vi "ArduPilot GCS.vi"() -> ()   [LabVIEW 8.6]
uses:
  user32.dll
  EventHandlerEnum.ctl
  Engines/SettingsEngine/SettingsEngineEnum.ctl
  EnumComm.ctl
  Engines/LogEngine/EnumLog.ctl
  Engines/SpeachEngine/EnumSpeak.ctl
panel:
  out "IMU":bool
  out "Climb Rate":dbl(knob) scale=-10.0..10.0 scale format="%#.2g"
  out "Mode":string
  out "WP":i32
  out "DistanceWP":i32 format="%.0f m"
  out "UAV Longitude":dbl format="%.6g°"
  out "UAV Latitude":dbl format="%.6g°"
  out "Throttle":i32(slide) scale=0.0..125.0
  out "Battery":dbl(slide) scale=0.0..10.0
  out "error outint comp manually":errorcluster
  out "error out clen-up":errorcluster
  in  "WebBrowser 2":refnum<k7>(container)
  in  "Heading":string="0"
  in  "Range":string="1000"
  in  "Tilt":string="0"
  in  "Send":bool
  in  "write buffer":string
  in  "Baud Rate":string(combo)="9600"
  in  "COM Port":refnum<visa-resource-name>
  out "Comm Status":bool
  in  "EARTHLib.IApplicationGE":refnum<k7>
  in  "EARTHLib.IKHInterface":refnum<k7>
  out "GPS fix":bool
  out "error out":errorcluster
  out "StatusMsg":string
  in  "Stop":bool
  in  "Tab Control":T1(tab)
  out "GndSpeed":i32(knob) scale=0.0..50.0
  out "AirSpeed":i32(knob) caption="Air Speed" scale=0.0..50.0
  out "Course   Bearing":cluster{i32, i32}(knob) scale=0.0..360.0 scale format="%.0f°"
  out "Altitude":cluster{i32, i32}(knob) scale=0.0..200.0
  out "Pitch":i32
  out "Roll":i32
  out "Roll Ind":cluster{i32, i32}(knob)={0, 180} scale=0.0..360.0
  out "Pitch-pic":picture
  in  "Zoom":u16(slide)=1000 scale=60000.0..1.0
  in  "Tilt":u8(slide) scale=0.0..90.0
  in  "Connect":bool
  in  "Baud Rate -M":string(combo)="9600"
  in  "COM Port -M":refnum<visa-resource-name>
  in  "kml write interval [s]":u32=1
  in  "Announcement interval [sec]":u32=30
  in  "Pan":i16(knob) scale=0.0..359.0
  out "IMU Performance data":string
  out "IMU health":i32
  out "Debug / Not Telemetry Data":string
  out "Raw Data":string
  # "%%%PWP:\t\t376322464,\t-1224913280,\t300,\nNWP:0,\t376321530,\t-1224913400,\t1200,***"
  # "Climb Rate"
  # "-122.491"
  # "37.6322"
  # "lon 122\nlat 37"
  # "meters"
  # "ALH"
  # "m / s"
  # "0"
  # "NOT USED"
  # "meters"
  # "meters"
  # "ALH"
  # "ALH"
  # "ALT"
  # "Gnd Speed"
  # "m/s"
  # "CRS"
  # "ASD"
  # "GSD"
  # "BER"
  # "AP port - manuall connection"
  # "To manually connect to AP serial port\nselect desired 'COM port' and 'Boud Rate' values\nand press 'Connect'"
  # "Google Earth Controls"
  # "Audio"
  # "N"
  # "(How often to update kml (GE) display)"
  # "Received"
  # "Set"
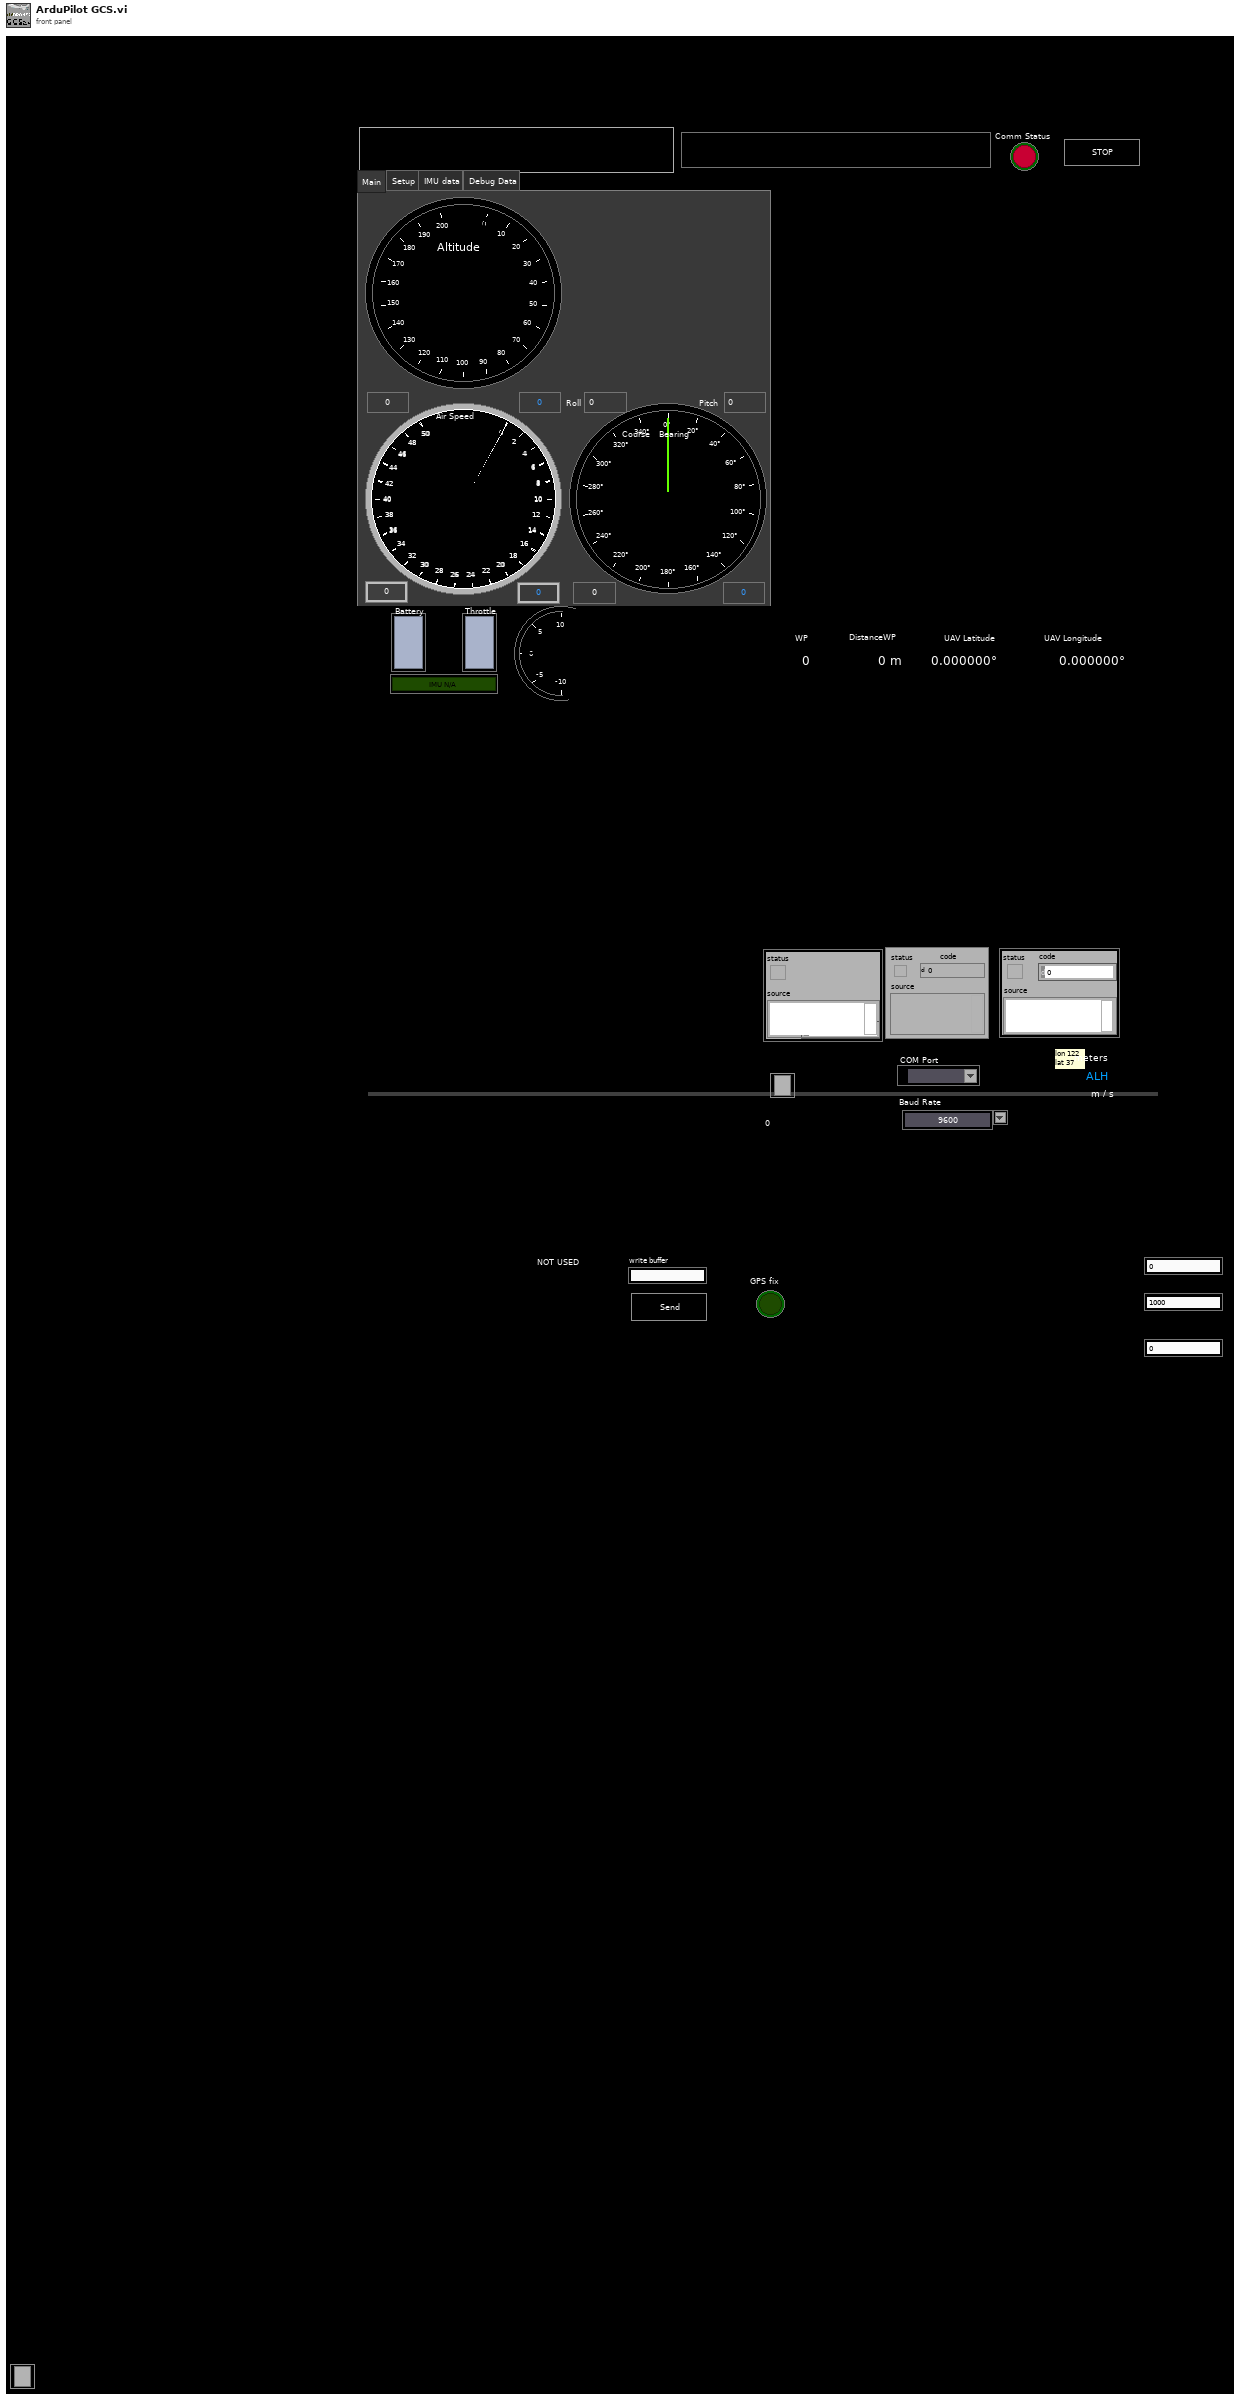
[diagram p1: front panel]
types:
  T1 = enum32{"Main", "Setup", "IMU data", "Debug Data"}
  T2 = typedef "EnumLog.ctl" = enum16{"Idle", "Log", "Init", "AddWP", "Stop", "CleanUp"}
  T3 = typedef "EnumComm.ctl" = enum16{"Read", "Idle", "Init", "InitComPort", "InitComPortManually", "Stop", "CleanUp", "Send"}
  T4 = typedef "EventHandlerEnum.ctl" = enum16{"Timeout", "Stop", "UpdateGEView", "UpdateCamData", "FPV_View_On", "UpdateIndicators"}
  T5 = typedef "EnumSpeak.ctl" = enum16{"Idle", "Init", "Speak", "Close"}
  T6 = cluster{"output number":i32, "output number":i32}
  T7 = typedef "SettingsEngineEnum.ctl" = enum16{"Init", "Load Settings from File", "Get Setting", "Set/Create Setting", "Save Settings to File"}
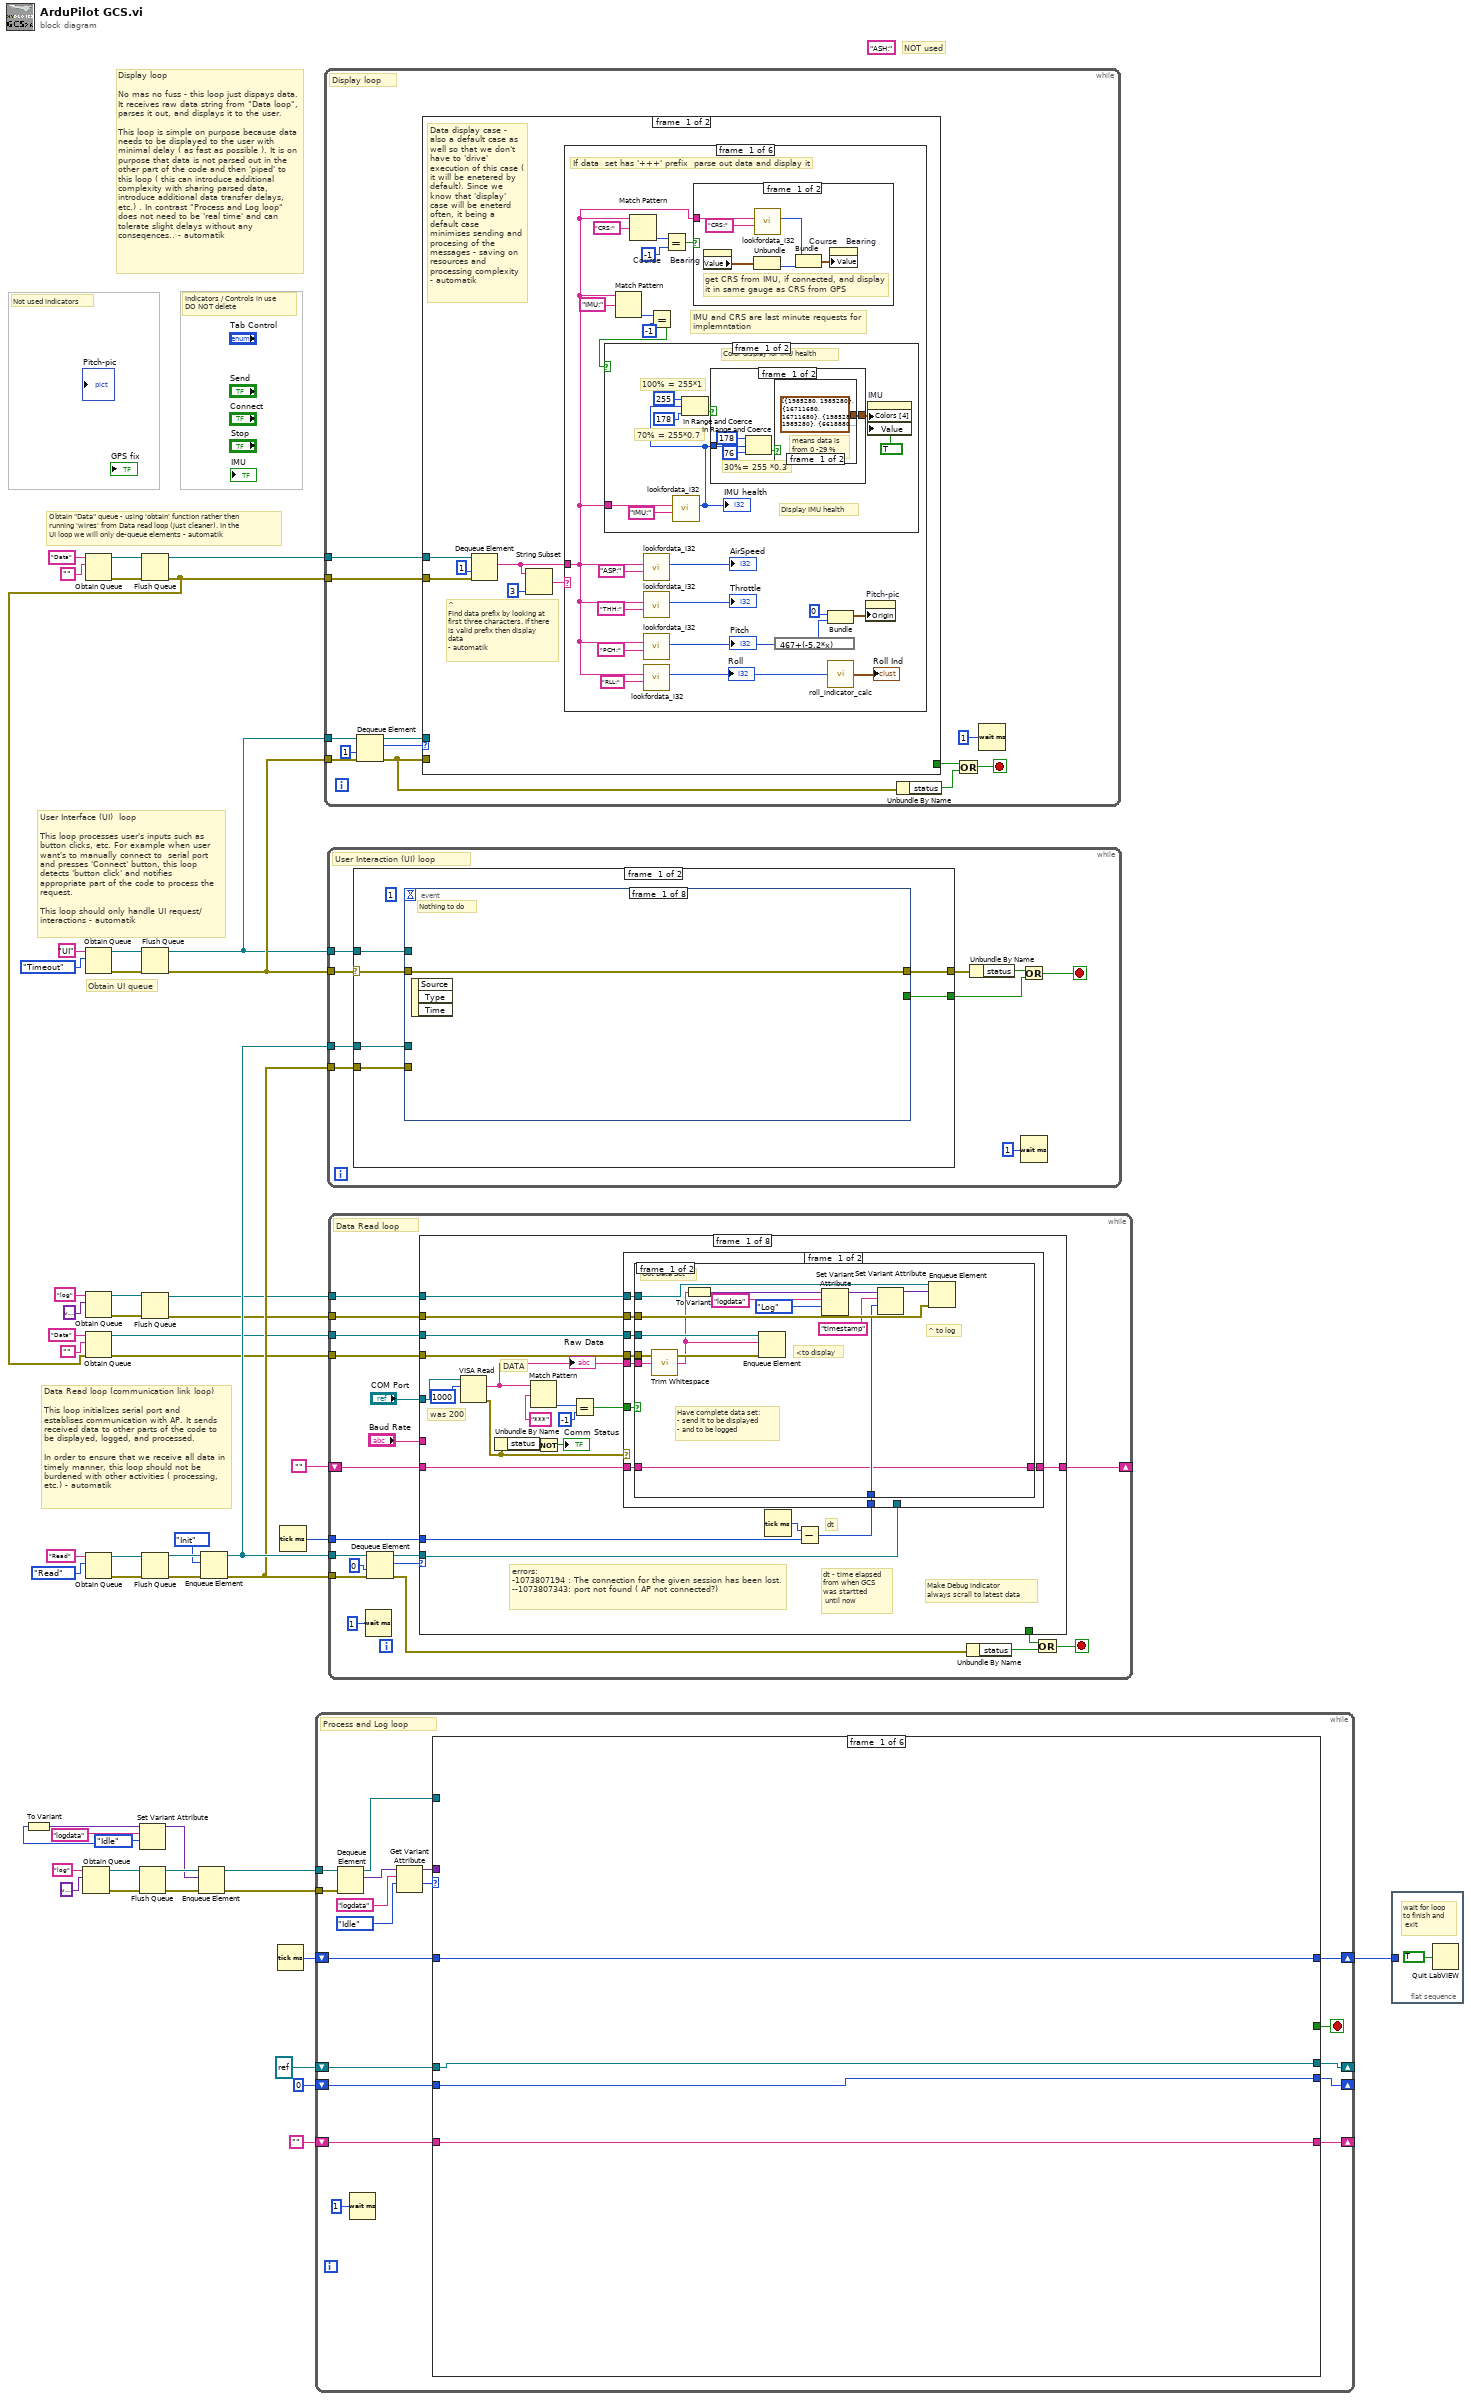
[diagram p0: block diagram]
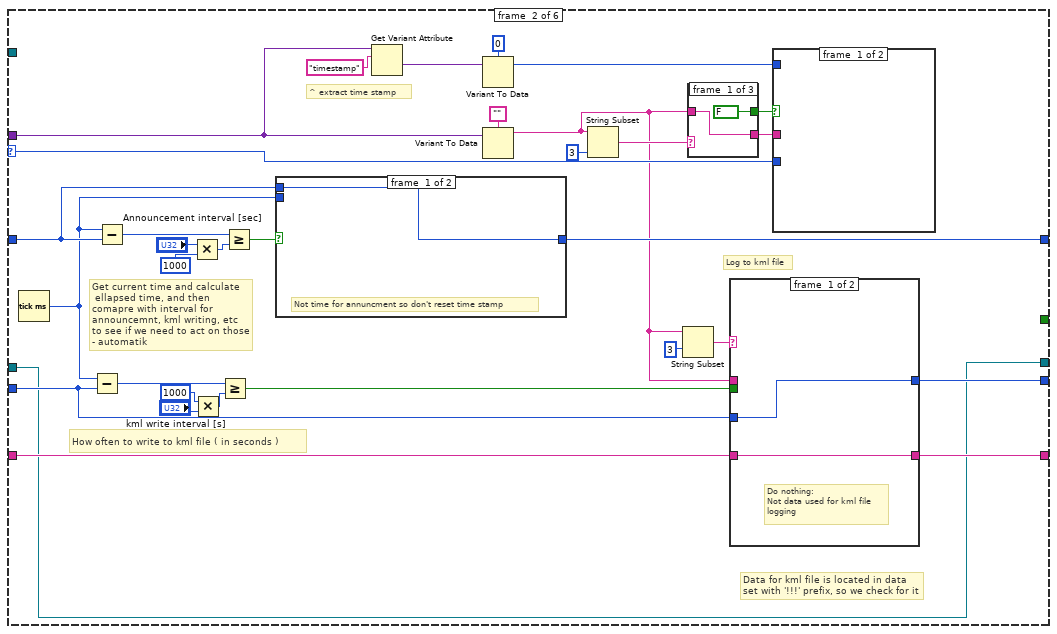
[diagram p2: hidden frame]
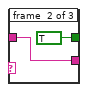
[diagram p3: hidden frame]
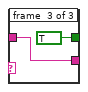
[diagram p4: hidden frame]
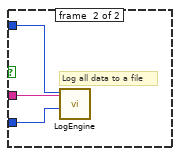
[diagram p5: hidden frame]
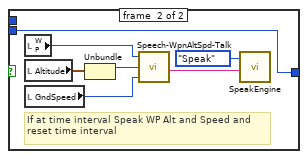
[diagram p6: hidden frame]
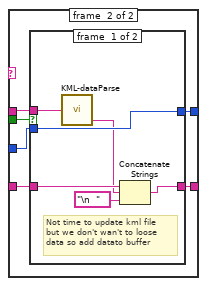
[diagram p7: hidden frame]
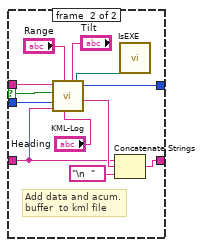
[diagram p8: hidden frame]
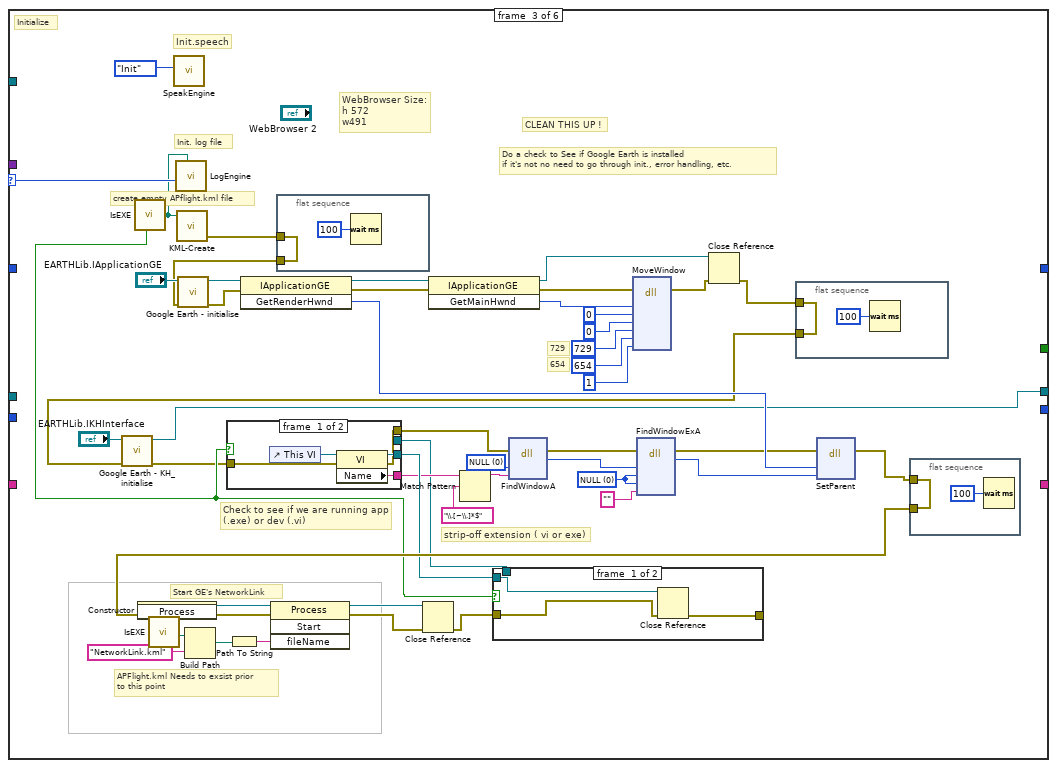
[diagram p9: hidden frame]
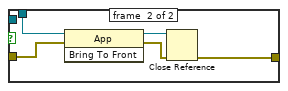
[diagram p10: hidden frame]
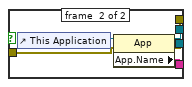
[diagram p11: hidden frame]
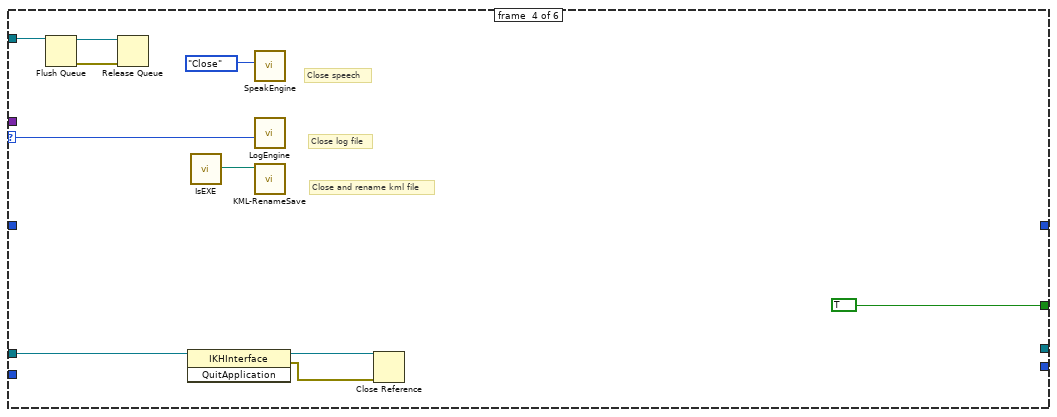
[diagram p12: hidden frame]
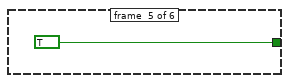
[diagram p13: hidden frame]
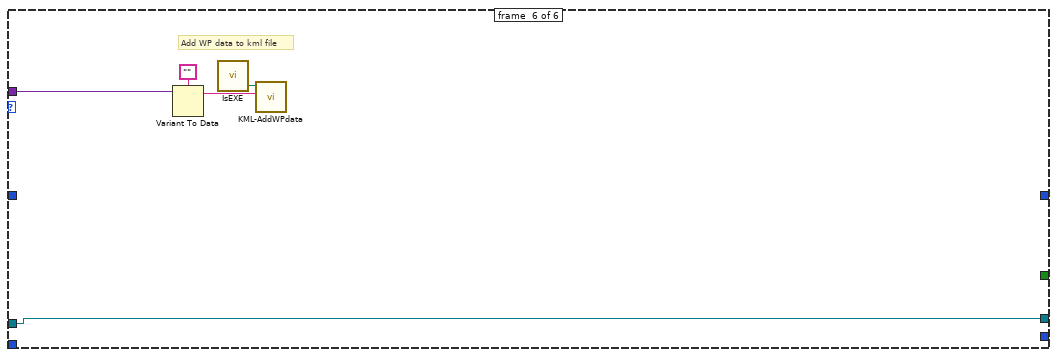
[diagram p14: hidden frame]
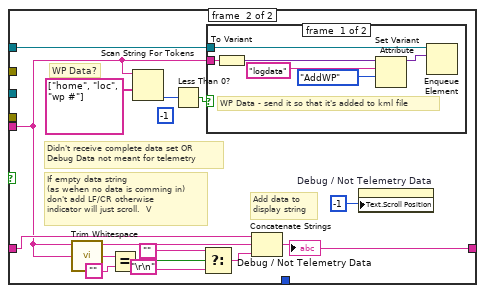
[diagram p15: hidden frame]
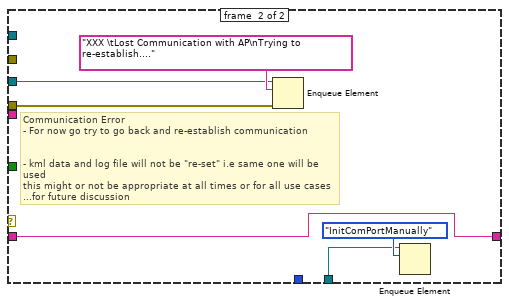
[diagram p17: hidden frame]
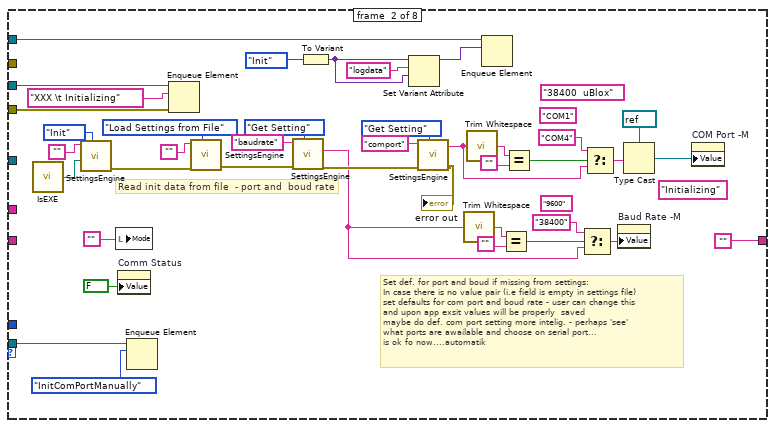
[diagram p18: hidden frame]
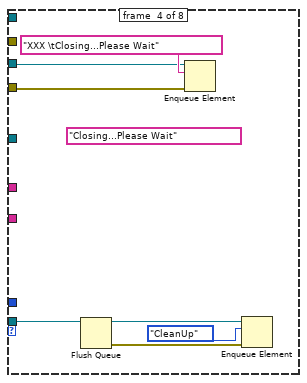
[diagram p20: hidden frame]
diagram:
  (unwired) "ASH:" ("regular expression")
  w12 = EnumLog."Idle" ("Log Enum")
  # "NOT used"
  # "Data Read loop (communication link loop)\n\nThis loop initializes serial port and establises communication with AP. It sends received data to other parts of the code to be displayed, logged, and processed.\n\nIn order to ensure that we receive all data in timely manner, this loop should not be burdened with other activities ( processing, etc.) - automatik"
  # "Obtain UI queue"
  # "User Interface (UI)  loop\n\nThis loop processes user's inputs such as button clicks, etc. For example when user want's to manually connect to  serial port and presses 'Connect' button, this loop detects 'button click' and notifies appropriate part of the code to process the request.\n\nThis loop should only handle UI request/ interactions - automatik"
  # "Obtain \"Data\" queue - using 'obtain' function rather then\nrunning 'wires' from Data read loop (just cleaner). In the\nUI loop we will only de-queue elements - automatik"
  # "Display loop\n\nNo mas no fuss - this loop just dispays data. It receives raw data string from \"Data loop\", parses it out, and displays it to the user. \n\nThis loop is simple on purpose because data needs to be displayed to the user with minimal delay ( as fast as possible ). It is on purpose that data is not parsed out in the other part of the code and then 'piped' to this loop ( this can introduce additional complexity with sharing parsed data, introduce additional data transfer delays, etc.) . In contrast \"Process and Log loop\"  does not need to be 'real time' and can tolerate slight delays without any conseqences.. - automatik"
  # "Indicators / Controls in use\nDO NOT delete"
  # "Not used indicators"
  n1 = To Variant(anything=w12) -> (Variant=w13:variant)
  n2 = Obtain Queue(name (unnamed)="log", element data type=variant ("variant")) -> (queue out=w19:refnum<queue>, error out=w7:errorcluster)  [unwired: 3 in, 1 out]
  n3 = Obtain Queue(name (unnamed)="Data", element data type="") -> (queue out=w29:refnum<queue>, error out=w27:errorcluster)  [unwired: 3 in, 1 out]
  n4 = Obtain Queue(name (unnamed)="UI", element data type=EventHandlerEnum."Timeout" ("Enum")) -> (queue out=w38:refnum<queue>, error out=w40:errorcluster)  [unwired: 3 in, 1 out]
  n5 = Obtain Queue(name (unnamed)="log", element data type=variant ("variant")) -> (queue out=w24:refnum<queue>, error out=w23:errorcluster)  [unwired: 3 in, 1 out]
  n6 = Obtain Queue(name (unnamed)="Read", element data type=EnumComm."Read" ("Comm Enum")) -> (queue out=w48:refnum<queue>, error out=w47:errorcluster)  [unwired: 3 in, 1 out]
  n7 = Set Variant Attribute(Variant=w13, name="logdata", value=w12) -> (Variant out=w11:variant)  [unwired: 1 in, 2 out]
  n8 = Flush Queue(queue=w19, error in (no error)=w7) -> (queue out=w16:refnum<queue>, error out=w5:errorcluster)  [unwired: 1 out]
  n9 = Flush Queue(queue=w29, error in (no error)=w27) -> (queue out=w28:refnum<queue>, error out=w26:errorcluster)  [unwired: 1 out]
  n10 = Obtain Queue(name (unnamed)="Data", element data type="", error in (no error)=w26) -> (queue out=w31:refnum<queue>, error out=w30:errorcluster)  [unwired: 2 in, 1 out]
  n11 = Flush Queue(queue=w38, error in (no error)=w40) -> (queue out=w37:refnum<queue>, error out=w39:errorcluster)  [unwired: 1 out]
  n12 = Flush Queue(queue=w24, error in (no error)=w23) -> (queue out=w22:refnum<queue>, error out=w21:errorcluster)  [unwired: 1 out]
  n13 = Flush Queue(queue=w48, error in (no error)=w47) -> (queue out=w46:refnum<queue>, error out=w45:errorcluster)  [unwired: 1 out]
  n14 = Enqueue Element(queue=w16, element=w11, error in (no error)=w5) -> (queue out=w15:refnum<queue>, error out=w4:errorcluster)  [unwired: 1 in, 1 out]
  n15 = Enqueue Element(queue=w46, element=EnumComm."Init" ("Comm Enum"), error in (no error)=w45) -> (queue out=w42:refnum<queue>, error out=w41:errorcluster)  [unwired: 1 in, 1 out]
  n16 = Tick Count (ms)() -> (millisecond timer value=w6:u32)
  n17 = Tick Count (ms)() -> (millisecond timer value=w10:u32)
  n18 = while {
    tunnel: w15 -> [w53]
    tunnel: w4 -> [w68]
    shift-right: [w61] -> _
    shift-left: "" -> [w60]
    shift-right: [w59] -> _
    shift-left: u32 0 ("millisecond timer value") -> [w58]
    shift-right: [w55] -> w2
    shift-left: w6 -> [w56]
    shift-right: [w52] -> _
    shift-left: refnum<k7> refnum ("Refnum Out") -> [w51]
    stop <- w63 stop-if-true
    # "Process and Log loop"
    n19 = Dequeue Element(queue=w53, error in (no error)=w68) -> (queue out=w54:refnum<queue>, element=w67:variant)  [unwired: 1 in, 2 out]
    n20 = Wait (ms)(milliseconds to wait=u32 1) -> ()  [unwired: 1 out]
    n21 = Get Variant Attribute(Variant=w67, name="logdata", default value (empty Variant)=EnumLog."Idle" ("Log Enum")) -> (duplicate Variant=w64:variant, value=w65:T2)  [unwired: 1 in, 2 out]
    n22 = case shown="\"Init\"" w65 {
      selector: w65 -> [_ w94 w193 w230 _ _]
      tunnel: w64 -> [_ w103 _ _ _ w236]
      tunnel: [_ _ _ TRUE ("x") TRUE ("x") _] -> w63
      tunnel: [w71 w97 _ _ _ _] -> w61
      tunnel: w60 -> [w71 w96 _ _ _ _]
      tunnel: [w72 w95 _ _ _ _] -> w59
      tunnel: w58 -> [w72 w93 _ _ _ _]
      tunnel: w56 -> [w70 w82 _ _ _ _]
      tunnel: [w70 w80 _ _ _ _] -> w55
      tunnel: w54 -> [_ _ _ w226 _ _]
      tunnel: [w69 w73 w151 _ _ w233] -> w52
      tunnel: w51 -> [w69 w73 _ w224 _ w233]
      frame #0 {
      }
      frame #1 {
        # "Get current time and calculate\n ellapsed time, and then comapre with interval for announcemnt, kml writing, etc to see if we need to act on those - automatik"
        # "Data for kml file is located in data\nset with '!!!' prefix, so we check for it"
        # "^ extract time stamp"
        # "Log to kml file"
        # "How often to write to kml file ( in seconds )"
        n23 = Tick Count (ms)() -> (millisecond timer value=w81:u32)
        n24 = Subtract(x=w81, y=w93) -> (x-y=w98:u32)
        n25 = Subtract(x=w81, y=w82) -> (x-y=w84:u32)
        n26 = Multiply(x="Announcement interval [sec]", y=u32 1000) -> (x*y=w85:u32)
        n27 = Multiply(x=u32 1000, y="kml write interval [s]") -> (x*y=w89:u32)
        n28 = Greater Or Equal?(x=w98, y=w89) -> (x >= y?=w92:bool)
        n29 = Greater Or Equal?(x=w84, y=w85) -> (x >= y?=w83:bool)
        n30 = case shown="True" w83 {
          tunnel: w82 -> [w114 _]
          tunnel: w81 -> [_ w116]
          tunnel: [w114 w116] -> w80
          frame #0 {
            # "Not time for annuncment so don't reset time stamp"
          }
          frame #1 {
            # "If at time interval Speak WP Alt and Speed and reset time interval"
            n31 = local read "WP"() -> (w120:i32)
            n32 = local read "Altitude"() -> (w119:cluster{i32, i32})
            n33 = local read "GndSpeed"() -> (w115:i32)
            n34 = Unbundle(w119) -> (w121:i32)  [unwired: 1 out]
            n35 = call "Speech-WpnAltSpd-Talk.vi"("Ground Speed"=w115, "Altitude"=w121, "Current WP"=w120) -> ("Text"=w118:string)
            n36 = call "SpeakEngine.vi"("Text to speak"=w118, "EnumSpeak"=EnumSpeak."Speak") -> ()  [unwired: 9 in, 1 out]
          }
        }
        n37 = Get Variant Attribute(Variant=w103, name="timestamp") -> (value=w101:variant)  [unwired: 2 in, 3 out]
        n38 = Variant To Data(Variant=w101, type=u32 0 ("x-y 2")) -> (data=w99:u32)  [unwired: 1 in, 1 out]
        n39 = Variant To Data(Variant=w103, type="") -> (data=w75:string)  [unwired: 1 in, 1 out]
        n40 = String Subset(string=w75, length (rest)=3 ("length (rest)")) -> (substring=w76:string)  [unwired: 1 in]
        n41 = String Subset(string=w75, length (rest)=3 ("length (rest)")) -> (substring=w90:string)  [unwired: 1 in]
        n42 = case shown="\"+++\"" w76 {
          tunnel: [w105 w107 w109] -> w79
          tunnel: [FALSE TRUE TRUE] -> w78
          tunnel: w75 -> [w105 w107 w109]
          frame #0 {
          }
          frame #1 {
          }
          frame #2 {
          }
        }
        n43 = case shown="\"!!!\"" w90 {
          tunnel: [w122 w129] -> w97
          tunnel: w96 -> [w122 w128]
          tunnel: [w123 w127] -> w95
          tunnel: w93 -> [w123 w126]
          tunnel: w92 -> [_ w124]
          tunnel: w75 -> [_ w125]
          frame #0 {
            # "Do nothing:\nNot data used for kml file\nlogging"
          }
          frame #1 {
            n44 = case shown="True" w124 {
              selector: w124 -> [_ w139]
              tunnel: [w132 w146] -> w129
              tunnel: w128 -> [w133 w143]
              tunnel: [w134 w142] -> w127
              tunnel: w126 -> [w134 w141]
              tunnel: w125 -> [w131 w140]
              frame #0 {
                # "Not time to update kml file\nbut we don't wan't to loose\ndata so add datato buffer"
                n45 = call "KML-dataParse.vi"("data in"=w131) -> ("Cur loc (out)"=w130:string)  [unwired: 1 in, 1 out]
                n46 = Concatenate Strings(w133, w130, "\n  " ("string")) -> (w132:string)
              }
              frame #1 {
                # "Add data and acum. \nbuffer  to kml file"
                n47 = call "IsEXE.vi"() -> ("path to vi or exe install\\data\\ dir"=w145:path)  [unwired: 10 out]
                n48 = call "KML-Log.vi"("path to vi or exe (in)"=w145, "Tilt"="Tilt", "Heading"="Heading", "Range"="Range", "Coords (in)"=w143, "TimerIN (sh)"=w141, "WriteToFile?"=w139, "data in"=w140) -> ("Cur loc (out)"=w144:string, "Timer OUT (sh)"=w142:u32)  [unwired: 2 in]
                n49 = Concatenate Strings(w143, w144, "\n  " ("string")) -> (w146:string)
              }
            }
          }
        }
        n50 = case shown="True" w78 {
          tunnel: w99 -> [_ w113]
          tunnel: w94 -> [_ w112]
          tunnel: w79 -> [_ w111]
          frame #0 {
          }
          frame #1 {
            # "Log all data to a file"
            n51 = call "LogEngine.vi"("Log Enum"=w112, "LogDataIN"=w111, "cumul time"=w113) -> ()  [unwired: 9 in]
          }
        }
      }
      frame #2 {
        w181 = 0 items=["NULL"]
        w190 = 0 items=["NULL"]
        # "CLEAN THIS UP !"
        # "strip-off extension ( vi or exe)"
        # "Check to see if we are running app\n(.exe) or dev (.vi)"
        # "Do a check to See if Google Earth is installed\nif it's not no need to go through init., error handling, etc."
        # "create empty APflight.kml file"
        # "WebBrowser Size:\nh 572\nw491"
        # "729"
        # "654"
        # "APFlight.kml Needs to exsist prior\nto this point"
        # "Start GE's NetworkLink"
        # "Init.speech"
        # "Init. log file"
        # "Initialize"
        n52 = call "Google Earth - KH_initialise.vi"("error in (no error)"=w168, "EARTHLib.IKHInterface"="EARTHLib.IKHInterface") -> ("error out"=w152:errorcluster, "Refnum Out"=w151:refnum<k7>)  [unwired: 8 out]
        n53 = call "IsEXE.vi"() -> ("path to vi or exe install\\data\\ dir"=w163:path, "is exe?"=w161:bool)  [unwired: 9 out]
        n54 = constructor class="Process"(error in=w164) -> (reference out=w170:refnum<k24>, error out=w169:errorcluster)  [unwired: 2 in, 1 out]
        n55 = call "IsEXE.vi"() -> ("path to vi or exe install\\data\\ dir"=w195:path)  [unwired: 10 out]
        n56 = call "SpeakEngine.vi"("EnumSpeak"=EnumSpeak."Init") -> ()  [unwired: 10 in, 1 out]
        n57 = call "LogEngine.vi"("dir path to file"=w163, "Log Enum"=w193) -> ()  [unwired: 10 in]
        n58 = call "KML-Create.vi"("path to vi or exe install\\data\\ dir"=w163) -> ("error out"=w167:errorcluster)  [unwired: 4 in]
        n59 = call "Google Earth - initialise.vi"("error in (no error)"=w166, "EARTHLib.IApplicationGE"="EARTHLib.IApplicationGE") -> ("error out"=w183:errorcluster, "Refnum Out"=w182:refnum<k7>)  [unwired: 8 out]
        n60 = Build Path(base path=w195, name or relative path="NetworkLink.kml") -> (appended path=w196:path)
        n61 = case shown="True" w161 {
          tunnel: [w210 w214] -> w158
          tunnel: [w209 _] -> w162
          tunnel: [_ w213] -> w153
          tunnel: w152 -> [w207 w212]
          tunnel: [w206 w211] -> w160
          frame #0 {
            n62 = control-ref of="This VI"() -> (w208:refnum<vi>)
            n63 = property class="VI"(reference=w208, error in=w207) -> (reference out=w209:refnum<vi>, error out=w206:errorcluster, "Name"=w210:string)
          }
          frame #1 {
            n64 = control-ref of="This Application"() -> (w215:refnum<vi>)
            n65 = property class="App"(reference=w215, error in=w212) -> (reference out=w213:refnum<vi>, error out=w211:errorcluster, "App.Name"=w214:string)
          }
        }
        n66 = Path To String(path=w196) -> (string=w192:string)
        n67 = invoke class="IApplicationGE" method="GetRenderHwnd"(reference=w182, error in=w183) -> (reference out=w179:refnum<k7>, error out=w178:errorcluster, "GetRenderHwnd"=w185:i32)  [unwired: 1 in]
        n68 = invoke class="Process" method="Start"(reference=w170, error in=w169, "fileName"=w192) -> (reference out=w150:refnum<k24>, error out=w149:errorcluster)  [unwired: 1 in, 2 out]
        n69 = flat-sequence {
          tunnel: w167 -> [w218]
          tunnel: [w218] -> w166
          frame #0 {
            n70 = Wait (ms)(milliseconds to wait=u32 100) -> ()  [unwired: 1 out]
          }
        }
        n71 = Close Reference(reference=w150, error in (no error)=w149) -> (error out=w148:errorcluster)
        n72 = invoke class="IApplicationGE" method="GetMainHwnd"(reference=w179, error in=w178) -> (reference out=w156:refnum<k7>, error out=w171:errorcluster, "GetMainHwnd"=w173:i32)  [unwired: 1 in]
        n73 = Match Pattern(string=w158, regular expression="\\.[~\\.]*$") -> (before substring=w157:string)  [unwired: 4 out]
        n74 = case shown="True" w161 {
          tunnel: w148 -> [w198 w204]
          tunnel: w162 -> [w199 _]
          tunnel: w153 -> [_ w202]
          tunnel: [w200 w205] -> _
          frame #0 {
            n75 = Close Reference(reference=w199, error in (no error)=w198) -> (error out=w200:errorcluster)
          }
          frame #1 {
            n76 = invoke class="App" method="Bring To Front"(reference=w202, error in=w204) -> (reference out=w201:refnum<vi>, error out=w203:errorcluster)  [unwired: 1 in, 1 out]
            n77 = Close Reference(reference=w201, error in (no error)=w203) -> (error out=w205:errorcluster)
          }
        }
        n78 = dll-call lib="user32.dll" fn="FindWindowA" label="FindWindow"(error in=w160, "lpszClassName"=w190, "lpszWindowName"=w157) -> (error out=w186:errorcluster, "hWnd"=w189:u32)  [unwired: 4 in, 1 out]
        n79 = dll-call lib="user32.dll" fn="MoveWindow"(error in=w171, "hWnd"=w173, "X"=u32 0, "Y"=0, "nWidth"=u32 729, "nHeight"=u32 654, "bRepaint"=u8 1) -> (error out=w155:errorcluster)  [unwired: 5 in, 5 out]
        n80 = dll-call lib="user32.dll" fn="FindWindowExA" label="Find Child"(error in=w186, "Parent HWND"=w189, "Child_After HWND"=w181, "lpszClassName"=w181, "lpszWindowName"="") -> (error out=w180:errorcluster, "hWnd"=w188:u32)  [unwired: 5 in, 2 out]
        n81 = Close Reference(reference=w156, error in (no error)=w155) -> (error out=w154:errorcluster)
        n82 = flat-sequence {
          tunnel: w154 -> [w220]
          tunnel: [w220] -> w168
          frame #0 {
            n83 = Wait (ms)(milliseconds to wait=u32 100) -> ()  [unwired: 1 out]
          }
        }
        n84 = dll-call lib="user32.dll" fn="SetParent" label="Set Parent"(error in=w180, "hWndChild"=w185, "hWndNewParent"=w188) -> (error out=w165:errorcluster)  [unwired: 4 in, 2 out]
        n85 = flat-sequence {
          tunnel: w165 -> [w216]
          tunnel: [w216] -> w164
          frame #0 {
            n86 = Wait (ms)(milliseconds to wait=u32 100) -> ()  [unwired: 1 out]
          }
        }
      }
      frame #3 {
        # "Close speech"
        # "Close and rename kml file"
        # "Close log file"
        n87 = Flush Queue(queue=w226) -> (queue out=w228:refnum<queue>, error out=w227:errorcluster)  [unwired: 1 in, 1 out]
        n88 = Release Queue(queue=w228, error in (no error)=w227) -> ()  [unwired: 1 in, 3 out]
        n89 = invoke class="IKHInterface" method="QuitApplication"(reference=w224) -> (reference out=w223:refnum<k7>, error out=w222:errorcluster)  [unwired: 2 in, 1 out]
        n90 = call "IsEXE.vi"() -> ("path to vi or exe install\\data\\ dir"=w225:path)  [unwired: 10 out]
        n91 = call "SpeakEngine.vi"("EnumSpeak"=EnumSpeak."Close") -> ()  [unwired: 10 in, 1 out]
        n92 = call "LogEngine.vi"("Log Enum"=w230) -> ()  [unwired: 11 in]
        n93 = call "KML-RenameSave.vi"("path to vi or exe install\\data\\ dir"=w225) -> ()  [unwired: 11 in]
        n94 = Close Reference(reference=w223, error in (no error)=w222) -> ()  [unwired: 1 out]
      }
      frame #4 {
      }
      frame #5 {
        # "Add WP data to kml file"
        n95 = Variant To Data(Variant=w236, type="") -> (data=w235:string)  [unwired: 1 in, 1 out]
        n96 = call "IsEXE.vi"() -> ("path to vi or exe install\\data\\ dir"=w234:path)  [unwired: 10 out]
        n97 = call "KML-AddWPdata.vi"("wp data in (raw)"=w235, "kml file dir path"=w234) -> ()  [unwired: 9 in, 1 out]
      }
    }
  }
  n98 = while {
    tunnel: w37 -> [w239]
    tunnel: w39 -> [w238]
    tunnel: w26 -> [w244]
    tunnel: w28 -> [w243]
    stop <- w247 stop-if-true
    # "Display loop"
    n99 = Dequeue Element(queue=w239, timeout in ms (-1)=1 ("timeout in ms (-1) 2"), error in (no error)=w238) -> (queue out=w240:refnum<queue>, element=w249:T4, error out=w242:errorcluster)  [unwired: 1 out]
    n100 = case shown="\"Timeout\", Default" w249 {
      tunnel: w242 -> [_ w346]
      tunnel: [_ TRUE ("x")] -> w248
      tunnel: w244 -> [w250 _]
      tunnel: w243 -> [w251 _]
      tunnel: w240 -> [_ w345]
      frame #0 {
        # "Data display case - also a default case as well so that we don't have to 'drive' execution of this case ( it will be enetered by default). Since we know that 'display' case will be eneterd often, it being a default case  minimises sending and procesing of the messages - saving on resources and processing complexity\n- automatik"
        # "^\nFind data prefix by looking at first three characters. If there is valid prefix then display data\n- automatik"
        n101 = Dequeue Element(queue=w251, timeout in ms (-1)=1, error in (no error)=w250) -> (element=w254:string)  [unwired: 3 out]
        n102 = String Subset(string=w254, length (rest)=3 ("length (rest)")) -> (substring=w253:string)  [unwired: 1 in]
        n103 = case shown="\"+++\"" w253 {
          tunnel: w254 -> [w259 w304 w334 w336 w343 _]
          frame #0 {
            # "IMU and CRS are last minute requests for \nimplemntation"
            # "If data  set has '+++' prefix  parse out data and display it"
            n104 = Match Pattern(string=w259, regular expression="IMU:" ("Header")) -> (offset past match=w262:i32)  [unwired: 1 in, 3 out]
            n105 = Match Pattern(string=w259, regular expression="CRS:" ("Header")) -> (offset past match=w266:i32)  [unwired: 1 in, 3 out]
            n106 = call "lookfordata_i32.vi"("string (in)"=w259, "Header"="ASP:" ("regular expression")) -> ("output number"=→"AirSpeed":i32)  [unwired: 4 in, 2 out]
            n107 = call "lookfordata_i32.vi"("string (in)"=w259, "Header"="THH:" ("regular expression")) -> ("output number"=→"Throttle":i32)  [unwired: 4 in, 2 out]
            n108 = call "lookfordata_i32.vi"("string (in)"=w259, "Header"="PCH:") -> ("output number"=w257:i32)  [unwired: 4 in, 2 out]
            "Pitch" <- w257
            n109 = call "lookfordata_i32.vi"("string (in)"=w259, "Header"="RLL:") -> ("output number"=w258:i32)  [unwired: 4 in, 2 out]
            "Roll" <- w258
            n110 = Equal?(x=w262, y=-1) -> (x = y?=w260:bool)
            n111 = case shown="False" w260 {
              tunnel: w259 -> [w278 _]
              frame #0 {
                # "Display IMU health"
                # "70% = 255*0.7"
                # "100% = 255*1"
                # "Color display for IMU health"
                n112 = call "lookfordata_i32.vi"("string (in)"=w278, "Header"="IMU:") -> ("output number"=w279:i32)  [unwired: 4 in, 2 out]
                "IMU health" <- w279
                n113 = In Range and Coerce(upper limit=u8 255, x=w279, lower limit=u8 178) -> (In Range?=w281:bool)  [unwired: 1 out]
                n114 = case shown="False" w281 {
                  tunnel: [w285 cluster{"Color Box":u32, "Color Box 2":u32}[] [{"Color Box"=1985280, "Color Box 2"=1985280}, {"Color Box"=40757, "Color Box 2"=40757}, {"Color Box"=1985280, "Color Box 2"=1985280}, {"Color Box"=6618880, "Color Box 2"=6618880}] ("Colors [4] 5")] -> w280
                  tunnel: w279 -> [w289 _]
                  frame #0 {
                    # "30%= 255 *0.3"
                    n115 = In Range and Coerce(upper limit=u8 178, x=w289, lower limit=u8 76) -> (In Range?=w286:bool)  [unwired: 1 out]
                    n116 = case shown="True" w286 {
                      tunnel: [cluster{"Color Box":u32, "Color Box 2":u32}[] [{"Color Box"=1985280, "Color Box 2"=1985280}, {"Color Box"=16711680, "Color Box 2"=16711680}, {"Color Box"=1985280, "Color Box 2"=1985280}, {"Color Box"=6618880, "Color Box 2"=6618880}] ("Colors [4] 5") cluster{"Color Box":u32, "Color Box 2":u32}[] [{"Color Box"=1985280, "Color Box 2"=1985280}, {"Color Box"=16774930, "Color Box 2"=16774930}, {"Color Box"=1985280, "Color Box 2"=1985280}, {"Color Box"=6618880, "Color Box 2"=6618880}] ("Colors [4] 5")] -> w285
                      frame #0 {
                        # "means data is\nfrom 0 -29 %"
                      }
                      frame #1 {
                      }
                    }
                  }
                  frame #1 {
                  }
                }
                n117 = property on="IMU" class="Bool (strict)"("Colors [4]"=w280, "Value"=TRUE ("IMU")) -> ()  [unwired: 2 in, 2 out]
              }
              frame #1 {
                # "No IMU health data"
              }
            }
            n118 = Equal?(x=w266, y=-1) -> (x = y?=w264:bool)
            n119 = case shown="False" w264 {
              tunnel: w259 -> [w297 _]
              frame #0 {
                # "get CRS from IMU, if connected, and display\nit in same gauge as CRS from GPS"
                n120 = property on="Course   Bearing" class="Knob (strict)"() -> ("Value"=w294:cluster{i32, i32})  [unwired: 2 in, 2 out]
                n121 = Unbundle(w294) -> (w293:i32)  [unwired: 1 out]
                n122 = call "lookfordata_i32.vi"("string (in)"=w297, "Header"="CRS:") -> ("output number"=w295:i32)  [unwired: 4 in, 2 out]
                n123 = Bundle("output number"=w295, w293) -> (w296:cluster{"output number":i32, i32})  [unwired: 1 in]
                n124 = property on="Course   Bearing" class="Knob (strict)"("Value"=w296) -> ()  [unwired: 2 in, 2 out]
              }
              frame #1 {
                # "No CRS from IMU"
              }
            }
            n125 = expression code="467+(-5.2*x)"(w257) -> (w270:i32)
            n126 = Bundle("Scrollbar 2"=0, "output number"=w270) -> (w271:cluster{"Scrollbar 2":i32, "output number":i32})  [unwired: 1 in]
            n127 = call "roll_indicator_calc.vi"("Roll (in)"=w258) -> ("Roll Indicator (out)"=→"Roll Ind":cluster{"Roll ctrl":i32, i32})  [unwired: 4 in]
            n128 = property on="Pitch-pic" class="Pict"("Origin"=w271) -> ()  [unwired: 2 in, 2 out]
          }
          frame #1 {
            # "lon 122\nlat 37"
            # "Extra sapce left here in\ncase we need to add things"
            # "If data  set has '!!!' prefix  parse out data and display it"
            # "was i16"
            n129 = call "lookfordata_i32.vi"("string (in)"=w304, "Header"="LAT:") -> ("output number"=w316:i32)  [unwired: 4 in, 2 out]
            n130 = call "lookfordata_i32.vi"("string (in)"=w304, "Header"="LON:") -> ("output number"=w312:i32)  [unwired: 4 in, 2 out]
            n131 = call "lookfordata_i32.vi"("string (in)"=w304, "Header"="ALT:" ("regular expression")) -> ("output number"=w300:i32)  [unwired: 4 in, 2 out]
            n132 = call "lookfordata_i32.vi"("string (in)"=w304, "Header"="ALH:" ("regular expression")) -> ("output number"=w299:i32)  [unwired: 4 in, 2 out]
            n133 = call "lookfordata_i32.vi"("string (in)"=w304, "Header"="CRS:") -> ("output number"=w303:i32)  [unwired: 4 in, 2 out]
            n134 = call "lookfordata_i32.vi"("string (in)"=w304, "Header"="BER:") -> ("output number"=w302:i32)  [unwired: 4 in, 2 out]
            n135 = call "lookfordata_i32.vi"("string (in)"=w304, "Header"="SPD:") -> ("output number"=→"GndSpeed":i32)  [unwired: 4 in, 2 out]
            n136 = call "lookfordata_i32.vi"("string (in)"=w304, "Header"="WPN:") -> ("output number"=→"WP":i32)  [unwired: 4 in, 2 out]
            n137 = call "lookfordata_i32.vi"("string (in)"=w304, "Header"="DST:") -> ("output number"=→"DistanceWP":i32)  [unwired: 4 in, 2 out]
            n138 = call "lookfordata_dbl.vi"("Header"="CRT:", "string (in)"=w304) -> ("output_dbl"=→"Climb Rate":dbl)  [unwired: 4 in, 1 out]
            n139 = call "lookfordata_dbl.vi"("Header"="BTV:", "string (in)"=w304) -> ("output_dbl"=→"Battery":dbl)  [unwired: 4 in, 1 out]
            n140 = To Double Precision Float(number=w316) -> (double precision float=w315:dbl)
            n141 = To Double Precision Float(number=w312) -> (double precision float=w313:dbl)
            n142 = Bundle("output number"=w300, "output number"=w299) -> (→"Altitude":T6)  [unwired: 1 out]
            n143 = Bundle("output number"=w303, "output number"=w302) -> (→"Course   Bearing":T6)  [unwired: 1 out]
            n144 = expression code="x/1000000"(w313) -> (→"UAV Longitude":dbl)
            n145 = expression code="x/1000000"(w315) -> (→"UAV Latitude":dbl)
          }
          frame #2 {
            # "If data  set has '###' prefix  parse out data and display it"
            n146 = Match Pattern(string=w334, regular expression="###") -> (after substring=w331:string)  [unwired: 1 in, 3 out]
            n147 = Match Pattern(string=w331, regular expression="***") -> (before substring=w329:string)  [unwired: 1 in, 3 out]
            n148 = Match Pattern(string=w329, regular expression="\t") -> (before substring=→"Mode":string)  [unwired: 1 in, 3 out]
          }
          frame #3 {
            # "If data  set has 'XXX' prefix  parse out data and display it"
            # "Look at better ways \n  for passing data to\nStatusMsg (I.e rewrite)"
            n149 = Match Pattern(string=w336, regular expression="XXX") -> (after substring=w339:string)  [unwired: 1 in, 3 out]
            n150 = Match Pattern(string=w339, regular expression="***") -> (before substring=w337:string)  [unwired: 1 in, 3 out]
            n151 = Match Pattern(string=w337, regular expression="\t") -> (after substring=→"StatusMsg":string)  [unwired: 1 in, 3 out]
          }
          frame #4 {
            # "If data  set has 'PPP' prefix  parse out data and display it"
            n152 = Match Pattern(string=w343, regular expression="PPP") -> (after substring=→"IMU Performance data":string)  [unwired: 1 in, 3 out]
          }
          frame #5 {
            # "Received data set:\n- does not have a valid prefix (bad data or incomplete data set)\n or \n- there is nothing to display\nor\n- data set has not been received yet so code has nothing to dispay"
          }
        }
      }
      frame #1 {
        # "User pressed STOP button:\n\n- Release UI queue\n- send \"True\" signal to exit the loop \n- clean-up things (if any)"
        n153 = Release Queue(queue=w345, error in (no error)=w346) -> ()  [unwired: 1 in, 3 out]
      }
    }
    n154 = Unbundle By Name(w242) -> ("status"=w246:bool)
    n155 = Or(x=w248, y=w246) -> (x .or. y?=w247:bool)
    n156 = Wait (ms)(milliseconds to wait=u32 1) -> ()  [unwired: 1 out]
  }
  n157 = while {
    tunnel: w37 -> [w356]
    tunnel: w39 -> [w351]
    tunnel: w42 -> [w350]
    tunnel: w41 -> [w349]
    stop <- w352 stop-if-true
    # "User Interaction (UI) loop"
    n158 = case shown="No Error" w351 {
      selector: w351 -> [w359 w416]
      tunnel: w356 -> [w362 _]
      tunnel: [w361 w416] -> w354
      tunnel: [w360 _] -> w353
      tunnel: w350 -> [w358 _]
      tunnel: w349 -> [w357 _]
      frame #0 {
        (unwired) 1
        n159 = event shown="[2] Application Instance Close" {
          selector: _ -> [_ _ _ _ _ _ _ _]
          dyn-events: _ -> [_ _ _ _ _ _ _ _]
          timeout: _ -> [_ _ _ _ _ _ _ _]
          tunnel: w362 -> [_ w367 w391 _ _ _ _ _]
          tunnel: w359 -> [w363 w369 w393 _ _ _ _ _]
          tunnel: [w363 w368 w392 _ _ _ _ _] -> w361
          tunnel: [_ w364 TRUE _ _ _ _ _] -> w360
          tunnel: w358 -> [_ w366 w390 w396 w404 _ _ _]
          tunnel: w357 -> [_ w365 w389 w395 w403 _ _ _]
          event #0 {
            # "Nothing to do"
            n160 = event-data() -> ()  [unwired: 1 in, 3 out]
          }
          event #1 {
            # "User pressed STOP button"
            # "User pressed STOP button\nso send message to all components\nthat we are stopping.\nWe don't want to relese queues here as there might be 'clean-up' activities in other loops.\n\nSend 'True' signal to exit UI loop ( we are done and are exiting app...)"
            n161 = event-data() -> ("NewVal"=w364:bool)  [unwired: 1 in, 5 out]
            n162 = case shown="True" w364 {
              tunnel: w369 -> [w370 w375]
              tunnel: [w370 w381] -> w368
              tunnel: w367 -> [_ w380]
              tunnel: w366 -> [_ w378]
              tunnel: w365 -> [_ w372]
              frame #0 {
              }
              frame #1 {
                # "Empty queues to ensure STOP case is acted upon and that there are no 'residual' msgs"
                n163 = Flush Queue(queue=w380, error in (no error)=w375) -> (queue out=w376:refnum<queue>, error out=w374:errorcluster)  [unwired: 1 out]
                n164 = Flush Queue(queue=w378, error in (no error)=w372) -> (queue out=w373:refnum<queue>, error out=w371:errorcluster)  [unwired: 1 out]
                n165 = Enqueue Element At Opposite End(queue=w376, element=EventHandlerEnum."Stop", error in (no error)=w374) -> (error out=w381:errorcluster)  [unwired: 1 in, 2 out]
                n166 = Enqueue Element At Opposite End(queue=w373, element=EnumComm."Stop" ("Comm Enum"), error in (no error)=w371) -> ()  [unwired: 1 in, 3 out]
              }
            }
          }
          event #2 {
            # "Empty queues to ensure this  case is acted upon and that there are no 'residual' msgs"
            # "User initiated App Close"
            # "User initated app close  so send message to all components\nthat we are stopping.\nWe don't want to relese queues here as there might be 'clean-up' activities in other loops.\n\nSend 'True' signal to exit UI loop ( we are done and are exiting app...)"
            n167 = event-data() -> ()  [unwired: 1 in, 2 out]
            n168 = Flush Queue(queue=w391, error in (no error)=w393) -> (queue out=w385:refnum<queue>, error out=w384:errorcluster)  [unwired: 1 out]
            n169 = Flush Queue(queue=w390, error in (no error)=w389) -> (queue out=w383:refnum<queue>, error out=w382:errorcluster)  [unwired: 1 out]
            n170 = Enqueue Element At Opposite End(queue=w385, element=EventHandlerEnum."Stop", error in (no error)=w384) -> (error out=w392:errorcluster)  [unwired: 1 in, 2 out]
            n171 = Enqueue Element At Opposite End(queue=w383, element=EnumComm."Stop" ("Comm Enum"), error in (no error)=w382) -> ()  [unwired: 1 in, 3 out]
          }
          event #3 {
            # "User changed COM port or baud rate and pressed 'Connect' button"
            # "If code is here it means that user changed value\nof comm port or baud rate, so we will flush all data \nfrom queue and go to reinitilize com port with new\nsettings"
            n172 = event-data() -> ("NewVal"=w394:bool)  [unwired: 1 in, 1 out]
            n173 = case shown="True" w394 {
              tunnel: w396 -> [_ w400]
              tunnel: w395 -> [_ w397]
              frame #0 {
                # "Get value of button press:\nIf 'False\" user released button ('up-click') - do nothing"
              }
              frame #1 {
                # "Get value of button press:\nIf 'True\" user pressed down on the button"
                n174 = Flush Queue(queue=w400, error in (no error)=w397) -> (queue out=w399:refnum<queue>, error out=w398:errorcluster)  [unwired: 1 out]
                n175 = Enqueue Element(queue=w399, element=EnumComm."InitComPortManually" ("Comm Enum"), error in (no error)=w398) -> ()  [unwired: 1 in, 3 out]
              }
            }
          }
          event #4 {
            # "Case NOT used \nright now"
            # "SENDING DATA TO AP COM PORT IS CURRENTLY NOT USED\nIt's here for custom debuging putposes"
            n176 = event-data() -> ("NewVal"=w402:bool)  [unwired: 1 in, 1 out]
            n177 = case shown="True" w402 {
              tunnel: w404 -> [_ w408]
              tunnel: w403 -> [_ w405]
              frame #0 {
                # "Get value of button press:\nIf 'False\" user released button ('up-click') - do nothing"
              }
              frame #1 {
                # "Send Data to AP"
                n178 = Flush Queue(queue=w408, error in (no error)=w405) -> (queue out=w407:refnum<queue>, error out=w406:errorcluster)  [unwired: 1 out]
                n179 = Enqueue Element(queue=w407, element=EnumComm."Send" ("Comm Enum"), error in (no error)=w406) -> ()  [unwired: 1 in, 3 out]
              }
            }
          }
          event #5 {
            n180 = event-data() -> ()  [unwired: 1 in, 1 out]
            n181 = Number To Decimal String(number="Zoom") -> (decimal integer string=w410:string)  [unwired: 1 in]
            n182 = property on="Range" class="Str"("Value"=w410) -> ()  [unwired: 2 in, 2 out]
          }
          event #6 {
            n183 = event-data() -> ()  [unwired: 1 in, 1 out]
            n184 = Number To Decimal String(number="Tilt") -> (decimal integer string=w412:string)  [unwired: 1 in]
            n185 = property on="Tilt" class="Str"("Value"=w412) -> ()  [unwired: 2 in, 2 out]
          }
          event #7 {
            n186 = event-data() -> ()  [unwired: 1 in, 1 out]
            n187 = Number To Decimal String(number="Pan") -> (decimal integer string=w414:string)  [unwired: 1 in]
            n188 = property on="Heading" class="Str"("Value"=w414) -> ()  [unwired: 2 in, 2 out]
          }
        }
      }
      frame #1 {
        # "Queue Error - will exit the loop"
      }
    }
    n189 = Unbundle By Name(w354) -> ("status"=w355:bool)
    n190 = Or(x=w355, y=w353) -> (x .or. y?=w352:bool)
    n191 = Wait (ms)(milliseconds to wait=u32 1) -> ()  [unwired: 1 out]
  }
  n192 = while {
    tunnel: w42 -> [w418]
    tunnel: w41 -> [w417]
    tunnel: w31 -> [w427]
    tunnel: w30 -> [w426]
    tunnel: w22 -> [w425]
    tunnel: w21 -> [w424]
    tunnel: w10 -> [w423]
    shift-right: [w420] -> _
    shift-left: "" -> [w419]
    stop <- w430 stop-if-true
    # "Data Read loop"
    n193 = Wait (ms)(milliseconds to wait=u32 1) -> ()  [unwired: 1 out]
    n194 = Dequeue Element(queue=w418, timeout in ms (-1)=0, error in (no error)=w417) -> (queue out=w421:refnum<queue>, element=w434:T3, error out=w428:errorcluster)  [unwired: 1 out]
    n195 = case shown="\"Read\", Default" w434 {
      tunnel: w421 -> [w436 w543 _ w550 w573 w598 w626 _]
      tunnel: "COM Port" -> [w454 _ _ _ w558 _ _ w628]
      tunnel: [_ _ _ _ TRUE ("x") _ _ _] -> w432
      tunnel: w427 -> [w453 w510 _ w546 w568 w583 w624 _]
      tunnel: w426 -> [w452 w509 _ w545 w567 w585 w623 _]
      tunnel: w425 -> [w451 w512 _ _ w556 _ _ _]
      tunnel: w424 -> [w450 _ _ _ _ _ _ _]
      tunnel: w423 -> [w449 _ _ _ _ _ _ _]
      tunnel: "Baud Rate" -> [_ _ _ _ w557 _ _ _]
      tunnel: [w442 "" _ _ _ _ _ _] -> w420
      tunnel: w419 -> [w441 _ _ _ _ _ _ _]
      frame #0 {
        # "errors:\n-1073807194 : The connection for the given session has been lost.\n--1073807343: port not found ( AP not connected?)"
        # "Make Debug indicator\nalways scrall to latest data"
        # "dt - time elapsed\nfrom when GCS\nwas startted\n until now"
        # "dt"
        # "DATA"
        # "was 200"
        n196 = VISA Read(VISA resource name=w454, byte count=u32 1000) -> (read buffer=w438:string, error out=w437:errorcluster)  [unwired: 1 in, 2 out]
        "Raw Data" <- w438
        n197 = Unbundle By Name(w437) -> ("status"=w440:bool)
        n198 = Match Pattern(string=w438, regular expression="***") -> (offset past match=w445:i32)  [unwired: 1 in, 3 out]
        n199 = Not(x=w440) -> (.not. x?=→"Comm Status":bool)
        n200 = Equal?(x=w445, y=-1) -> (x = y?=w443:bool)
        n201 = Tick Count (ms)() -> (millisecond timer value=w448:u32)
        n202 = Subtract(x=w448, y=w449) -> (x-y=w447:u32)
        n203 = case shown="No Error" w437 {
          tunnel: w453 -> [w464 w501]
          tunnel: w452 -> [w463 w500]
          tunnel: w451 -> [w462 _]
          tunnel: w450 -> [w461 _]
          tunnel: w447 -> [w460 _]
          tunnel: w443 -> [w459 _]
          tunnel: [w458 w499] -> w442
          tunnel: w441 -> [w457 w499]
          tunnel: w438 -> [w456 _]
          tunnel: w436 -> [_ w503]
          frame #0 {
            n204 = case shown="False" w459 {
              tunnel: w464 -> [w478 _]
              tunnel: w463 -> [w477 _]
              tunnel: w462 -> [w476 w483]
              tunnel: w461 -> [w475 _]
              tunnel: w460 -> [w468 _]
              tunnel: w456 -> [w467 w480]
              tunnel: [w465 w491] -> w458
              tunnel: w457 -> [w465 w492]
              frame #0 {
                # "Have complete data set:\n- send it to be displayed\n- and to be logged"
                # "Got Data Set"
                # "^ to log"
                # "<to display"
                n205 = call <vilib>:"Trim Whitespace.vi"("string"=w467) -> ("trimmed string"=w466:string)  [unwired: 1 in]
                n206 = To Variant(anything=w466) -> (Variant=w473:variant)
                n207 = Enqueue Element(queue=w478, element=w466, error in (no error)=w477) -> ()  [unwired: 1 in, 3 out]
                n208 = Set Variant Attribute(Variant=w473, name="logdata", value=EnumLog."Log" ("Log Enum")) -> (Variant out=w471:variant)  [unwired: 1 in, 2 out]
                n209 = Set Variant Attribute(Variant=w471, name="timestamp", value=w468) -> (Variant out=w469:variant)  [unwired: 1 in, 2 out]
                n210 = Enqueue Element(queue=w476, element=w469, error in (no error)=w475) -> ()  [unwired: 1 in, 3 out]
              }
              frame #1 {
                (unwired) -1 ("y")
                # "Didn't receive complete data set OR\nDebug Data not meant for telemetry"
                # "WP Data?"
                # "Add data to \ndisplay string"
                # "If empty data string \n(as wehen no data is comming in)\ndon't add LF/CR otherwise \nindicator will just scroll.  V"
                n211 = call <vilib>:"Trim Whitespace.vi"("string"=w480) -> ("trimmed string"=w490:string)  [unwired: 1 in]
                n212 = Equal?(x=w490, y="") -> (x = y?=w488:bool)
                n213 = Scan String For Tokens(7:string[] ["home", "loc", "wp #"] ("operators (none)"), 9:w480) -> (0:w479:i32)  [unwired: 4 in, 3 out]
                n214 = Less Than 0?(x=w479) -> (x < 0?=w482:bool)
                n215 = Select(t="", s=w488, f="\r\n") -> (s? t:f=w486:string)
                n216 = case shown="False" w482 {
                  tunnel: w483 -> [w495 _]
                  tunnel: w480 -> [w493 _]
                  frame #0 {
                    # "WP Data - send it so that it's added to kml file"
                    n217 = To Variant(anything=w493) -> (Variant=w497:variant)
                    n218 = Set Variant Attribute(Variant=w497, name="logdata", value=EnumLog."AddWP" ("Log Enum")) -> (Variant out=w494:variant)  [unwired: 1 in, 2 out]
                    n219 = Enqueue Element(queue=w495, element=w494) -> ()  [unwired: 2 in, 3 out]
                  }
                  frame #1 {
                  }
                }
                n220 = Concatenate Strings(w492, w480, w486) -> (w491:string)
                "Debug / Not Telemetry Data" <- w491
                n221 = property on="Debug / Not Telemetry Data" class="Str"("Text.Scroll Position"=-1) -> ()  [unwired: 2 in, 2 out]
              }
            }
          }
          frame #1 {
            # "Communication Error\n- For now go try to go back and re-establish communication\n\n\n- kml data and log file will not be \"re-set\" i.e same one will be used\nthis might or not be appropriate at all times or for all use cases\n...for future discussion"
            n222 = Enqueue Element(queue=w501, element="XXX \tLost Communication with AP\nTrying to re-establish...." ("Setting Name"), error in (no error)=w500) -> ()  [unwired: 1 in, 3 out]
            n223 = Enqueue Element(queue=w503, element=EnumComm."InitComPortManually" ("Comm Enum")) -> ()  [unwired: 2 in, 3 out]
          }
        }
      }
      frame #1 {
        (unwired) "Initializing" ("Setting Name")
        (unwired) "9600" ("t")
        (unwired) "COM1" ("t")
        (unwired) "38400  uBlox" ("Baud Rate 2")
        # "Set def. for port and boud if missing from settings:\nIn case there is no value pair (i.e field is empty in settings file)\nset defaults for com port and boud rate - user can change this\nand upon app exsit values will be properly  saved\nmaybe do def. com port setting more intelig. - perhaps 'see'\nwhat ports are awailable and choose on serial port...\nis ok fo now....automatik"
        # "Read init data from file  - port and  boud rate"
        n224 = call "IsEXE.vi"() -> ("path to vi or exe install\\data\\ dir"=w507:path)  [unwired: 10 out]
        n225 = call "SettingsEngine.vi"("Enum"=SettingsEngineEnum."Init", "Dir for Settings File"=w507, "Setting Name"="") -> ("error out"=w541:errorcluster)  [unwired: 7 in, 1 out]
        n226 = local write "Mode"("") -> ()
        n227 = property on="Comm Status" class="Bool (strict)"("Value"=FALSE ("Comm")) -> ()  [unwired: 2 in, 2 out]
        n228 = Enqueue Element(queue=w543, element=EnumComm."InitComPortManually" ("Comm Enum")) -> ()  [unwired: 2 in, 3 out]
        n229 = Enqueue Element(queue=w510, element="XXX \t Initializing" ("Setting Name"), error in (no error)=w509) -> ()  [unwired: 1 in, 3 out]
        n230 = call "SettingsEngine.vi"("Enum"=SettingsEngineEnum."Load Settings from File", "error in"=w541, "Setting Name"="") -> ("error out"=w540:errorcluster)  [unwired: 7 in, 1 out]
        n231 = call "SettingsEngine.vi"("Enum"=SettingsEngineEnum."Get Setting", "error in"=w540, "Setting Name"="baudrate") -> ("error out"=w539:errorcluster, "Setting Value"=w526:string)  [unwired: 7 in]
        n232 = To Variant(anything=EnumLog."Init" ("Log Enum")) -> (Variant=w514:variant)
        n233 = Set Variant Attribute(Variant=w514, name="logdata", value=w514) -> (Variant out=w513:variant)  [unwired: 1 in, 2 out]
        n234 = call "SettingsEngine.vi"("Enum"=SettingsEngineEnum."Get Setting", "error in"=w539, "Setting Name"="comport") -> ("error out"=→"error out":errorcluster, "Setting Value"=w521:string)  [unwired: 7 in]
        n235 = call <vilib>:"Trim Whitespace.vi"("string"=w526) -> ("trimmed string"=w529:string)  [unwired: 1 in]
        n236 = call <vilib>:"Trim Whitespace.vi"("string"=w521) -> ("trimmed string"=w524:string)  [unwired: 1 in]
        n237 = Enqueue Element(queue=w512, element=w513) -> ()  [unwired: 2 in, 3 out]
        n238 = Equal?(x=w529, y="") -> (x = y?=w527:bool)
        n239 = Equal?(x=w524, y="") -> (x = y?=w522:bool)
        n240 = Select(t="38400", s=w527, f=w526) -> (s? t:f=w525:string)
        n241 = Select(t="COM4", s=w522, f=w521) -> (s? t:f=w520:string)
        n242 = property on="Baud Rate -M" class="CmbBox"("Value"=w525) -> ()  [unwired: 2 in, 2 out]
        n243 = Type Cast(type=refnum<visa-resource-name> refnum ("VISA resource name"), x=w520) -> (*(type *) &x=w530:refnum<visa-resource-name>)
        n244 = property on="COM Port -M" class="VISAName"("Value"=w530) -> ()  [unwired: 2 in, 2 out]
      }
      frame #2 {
        # "NOT USED now\n( it was used for auto detection\nof AP com port...)"
      }
      frame #3 {
        (unwired) "Closing...Please Wait" ("Setting Name")
        n245 = Flush Queue(queue=w550) -> (queue out=w549:refnum<queue>, error out=w548:errorcluster)  [unwired: 1 in, 1 out]
        n246 = Enqueue Element(queue=w546, element="XXX \tClosing...Please Wait" ("Setting Name"), error in (no error)=w545) -> ()  [unwired: 1 in, 3 out]
        n247 = Enqueue Element(queue=w549, element=EnumComm."CleanUp" ("Comm Enum"), error in (no error)=w548) -> ()  [unwired: 1 in, 3 out]
      }
      frame #4 {
        n248 = Flush Queue(queue=w568, error in (no error)=w567) -> (queue out=w570:refnum<queue>, error out=w569:errorcluster)  [unwired: 1 out]
        n249 = Flush Queue(queue=w573) -> (queue out=w572:refnum<queue>, error out=w571:errorcluster)  [unwired: 1 in, 1 out]
        n250 = Release Queue(queue=w570, error in (no error)=w569) -> (error out=w552:errorcluster)  [unwired: 1 in, 2 out]
        n251 = call "SettingsEngine.vi"("Enum"=SettingsEngineEnum."Set/Create Setting", "New Setting Value"=w558, "Setting Name"="comport") -> ("error out"=w564:errorcluster)  [unwired: 7 in, 1 out]
        n252 = Release Queue(queue=w572, error in (no error)=w571) -> (error out=w555:errorcluster)  [unwired: 1 in, 2 out]
        n253 = call "SettingsEngine.vi"("Enum"=SettingsEngineEnum."Set/Create Setting", "error in"=w564, "New Setting Value"=w557, "Setting Name"="baudrate") -> ("error out"=w559:errorcluster)  [unwired: 6 in, 1 out]
        n254 = VISA Flush I/O Buffer(VISA resource name=w558) -> (VISA resource name out=w576:refnum<visa-resource-name>, error out=w575:errorcluster)  [unwired: 1 in, 1 out]
        n255 = VISA Close(VISA resource name=w576, error in (no error)=w575) -> (error out=w554:errorcluster)
        "error out clen-up" <- w554
        n256 = call "SettingsEngine.vi"("Enum"=SettingsEngineEnum."Save Settings to File", "error in"=w559, "Setting Name"="a") -> ("error out"=w553:errorcluster)  [unwired: 7 in, 1 out]
        n257 = flat-sequence {
          tunnel: w556 -> [w577]
          tunnel: w555 -> [_]
          tunnel: w554 -> [_]
          tunnel: w553 -> [_]
          tunnel: w552 -> [_]
          frame #0 {
            # "Once everything finishes\nsend stop to log loop\n\n- could of used merge-errors\nbut didn't because I didn't\nwant to pass potential errors\nto logdata queue"
            n258 = To Variant(anything=EnumLog."Stop" ("Log Enum")) -> (Variant=w578:variant)
            n259 = Set Variant Attribute(Variant=w578, name="logdata", value=w578) -> (Variant out=w579:variant)  [unwired: 1 in, 2 out]
            n260 = Enqueue Element(queue=w577, element=w579) -> ()  [unwired: 2 in, 3 out]
          }
        }
      }
      frame #5 {
        w601 = u16 10 items=["1.0", "1.5", "2.0"] ("stop bits (10: 1 bit)")
        # "use \\r (0xD) as a terminator"
        n261 = Flush Queue(queue=w583, error in (no error)=w585) -> (queue out=w582:refnum<queue>, error out=w584:errorcluster)  [unwired: 1 out]
        n262 = VISA Open(duplicate session (F)=FALSE, VISA resource name="COM Port -M") -> (VISA resource name=w592:refnum<visa-resource-name>, error out=w591:errorcluster)  [unwired: 3 in]
        n263 = Decimal String To Number(string="Baud Rate -M") -> (number=w600:i32)  [unwired: 3 out]
        n264 = Flush Queue(queue=w598) -> (queue out=w596:refnum<queue>)  [unwired: 1 in, 2 out]
        n265 = Wait (ms)(milliseconds to wait=u32 10) -> ()  [unwired: 1 out]
        n266 = To Unsigned Long Integer(number=w600) -> (unsigned 32bit integer=w599:u32)
        n267 = call "VISA Configure Serial Port (Serial Instr).vi"("VISA resource name"=w592, "timeout (10sec)"=u32 2000, "termination char\n(0xA = '\\n' = LF)"=u8 13 ("termination char\n(0xA = '\\n' = LF)"), "Enable Termination\nChar (T)"=TRUE ("Enable Termination\nChar (T)"), "baud rate (9600)"=w599, "data bits (8)"=u16 8, "parity (0:none)"=enum16{"None", "Odd", "Even", "Mark", "Space"}."None", "error in (no error)"=w591, "stop bits (10: 1 bit)"=w601) -> ("VISA resource name out"=w593:refnum<visa-resource-name>, "error out"=w590:errorcluster)  [unwired: 5 in]
        n268 = case shown="No Error" w590 {
          selector: w590 -> [_ w615]
          tunnel: w596 -> [w612 w620]
          tunnel: w593 -> [w611 w619]
          tunnel: "Baud Rate -M" -> [w610 _]
          tunnel: [w609 w618] -> w588
          tunnel: w582 -> [w609 w618]
          tunnel: w584 -> [w608 w617]
          tunnel: [w608 w617] -> w589
          tunnel: ["XXX\tGCS Port Set" ("Setting Name") "XXX\tCould not set AP Com Port...\nis AP ON?)" ("Setting Name")] -> w587
          frame #0 {
            (unwired) "GCS Port Set" ("Setting Name")
            # "Communication established\nwith AP:\n-go to read data\n-init. proc.  and logging\n-display msg to user"
            # "Send msg to initialize data processing and logging\n(WAS here - moved)"
            n269 = local write "Baud Rate"(w610) -> ()
            n270 = local write "COM Port"(w611) -> ()
            n271 = Enqueue Element(queue=w612, element=EnumComm."Read" ("Comm Enum")) -> ()  [unwired: 2 in, 3 out]
          }
          frame #1 {
            # "Error - try connecting again"
            n272 = VISA Close(VISA resource name=w619, error in (no error)=w615) -> (error out=→"error outint comp manually":errorcluster)
            n273 = Enqueue Element(queue=w620, element=EnumComm."InitComPortManually" ("Comm Enum")) -> ()  [unwired: 2 in, 3 out]
          }
        }
        n274 = Enqueue Element(queue=w588, element=w587, error in (no error)=w589) -> ()  [unwired: 1 in, 3 out]
      }
      frame #6 {
        n275 = Enqueue Element(queue=w626, element=EnumComm."Idle" ("Comm Enum")) -> ()  [unwired: 2 in, 3 out]
        n276 = Enqueue Element(queue=w624, element="XXX\tCould not set AP Port...Try again ( is AP ON?)" ("Setting Name"), error in (no error)=w623) -> ()  [unwired: 1 in, 3 out]
      }
      frame #7 {
        (unwired) "SendingData" ("Setting Name")
        n277 = VISA Write(VISA resource name=w628, write buffer="write buffer") -> ()  [unwired: 1 in, 3 out]
      }
    }
    n278 = Unbundle By Name(w428) -> ("status"=w431:bool)
    n279 = Or(x=w432, y=w431) -> (x .or. y?=w430:bool)
  }
  n280 = flat-sequence {
    tunnel: w2 -> [_]
    frame #0 {
      # "wait for loop\nto finish and\n exit"
      n281 = Quit LabVIEW(quit? (T)=TRUE) -> ()
    }
  }
